vi "XYZ-BC.vi"(5 "加速度":dbl=600.0, 7 "最高速":dbl=1250.0, 8 "Error In":errorcluster, 9 "校正微動位置":enum16{"雙邊", "オ", "右", "相反"}(ring), 11 "X-Y-Z移動":dbl[](array[numeric])=[0.0, 0.0, 0.0]) -> (0 "Error Out":errorcluster)   [LabVIEW 2019]
uses:
  <vilib>/Platform/TimedLoop/XDataNode/timing_clust.ctl
  <vilib>/Platform/TimedLoop/XDataNode/nitl_modes.ctl
  <vilib>/Platform/TimedLoop/XDataNode/wakeup.ctl
  <vilib>/platform/TimedLoop/XDataNode/XDataNode.xnode
  <vilib>/Platform/TimedLoop/XDataNode/XDNodeRunTimeDep.lvlib
panel:
  in  "Stop":bool
  out "三角形?":bool
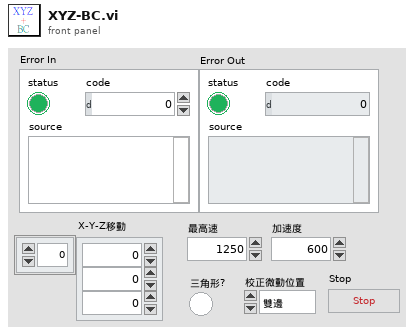
[diagram p1: front panel]
types:
  T1 = typedef "XDNodeRunTimeDep.lvlib/timing_clust.ctl" = cluster{"Expected End [f-1]":u64, "Actual End [f-1]":u64, "Finished Late? [f-1]":bool, "Expected End [i-1]":u64, "Actual End [i-1]":u64, "Finished Late? [i-1]":bool, "Expected Start [i]":u64, "Actual Start [i]":u64, "Expected Start [f]":u64, "Actual Start [f]":u64, "Source Name":string, "Structure Name":string, "Period":i64, "Deadline":i64, "Offset":i64, "Start":i64, "Priority":i32, "Timeout":i32, "Mode":T2, "Wakeup Reason":T3, "Error":errorcluster, "Source Type":string, "Secondary Source Type":string, "Global End Time":u64, "Global Start Time":u64, "Frame Duration":u64, "Iteration Duration":u64, "Assigned CPU":i32, "I/O Scan Engine Mode":u32}
  T2 = typedef "XDNodeRunTimeDep.lvlib/nitl_modes.ctl" = enum32{"No Change", "Process missed periods, maintain original phase", "Discard missed periods, maintain original phase", "Process missed periods, ignore original phase", "Discard missed periods, ignore original phase"}
  T3 = typedef "XDNodeRunTimeDep.lvlib/wakeup.ctl" = enum32{"Normal", "Aborted", "Asynchronous wakeup", "Timing source error", "Timed loop error", "Timeout"}
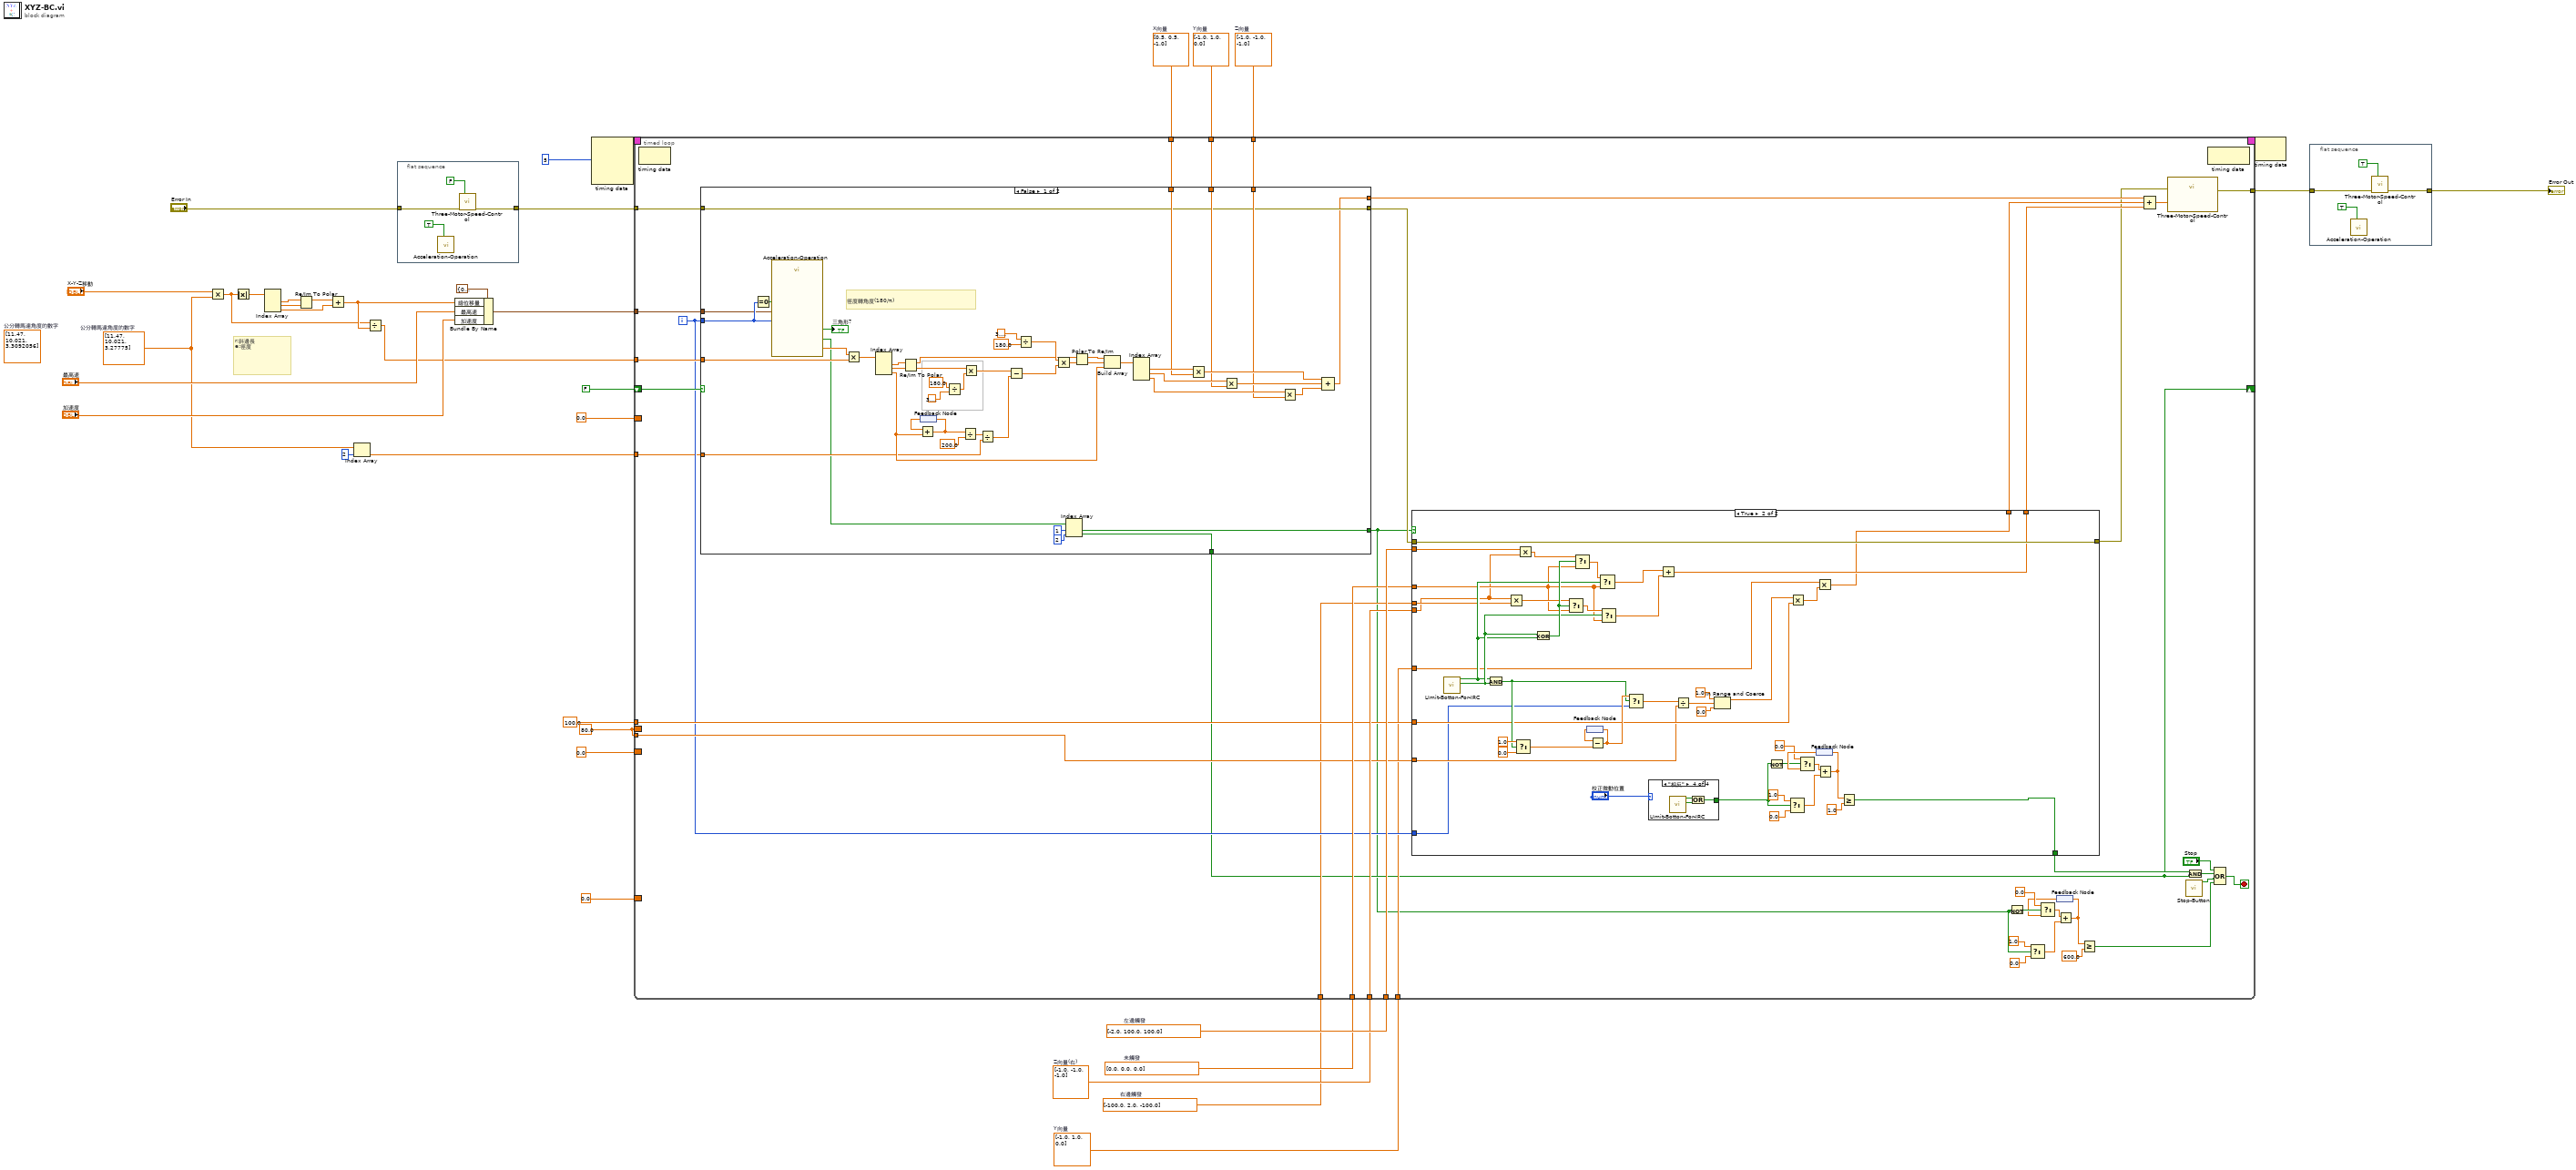
[diagram p0: block diagram]
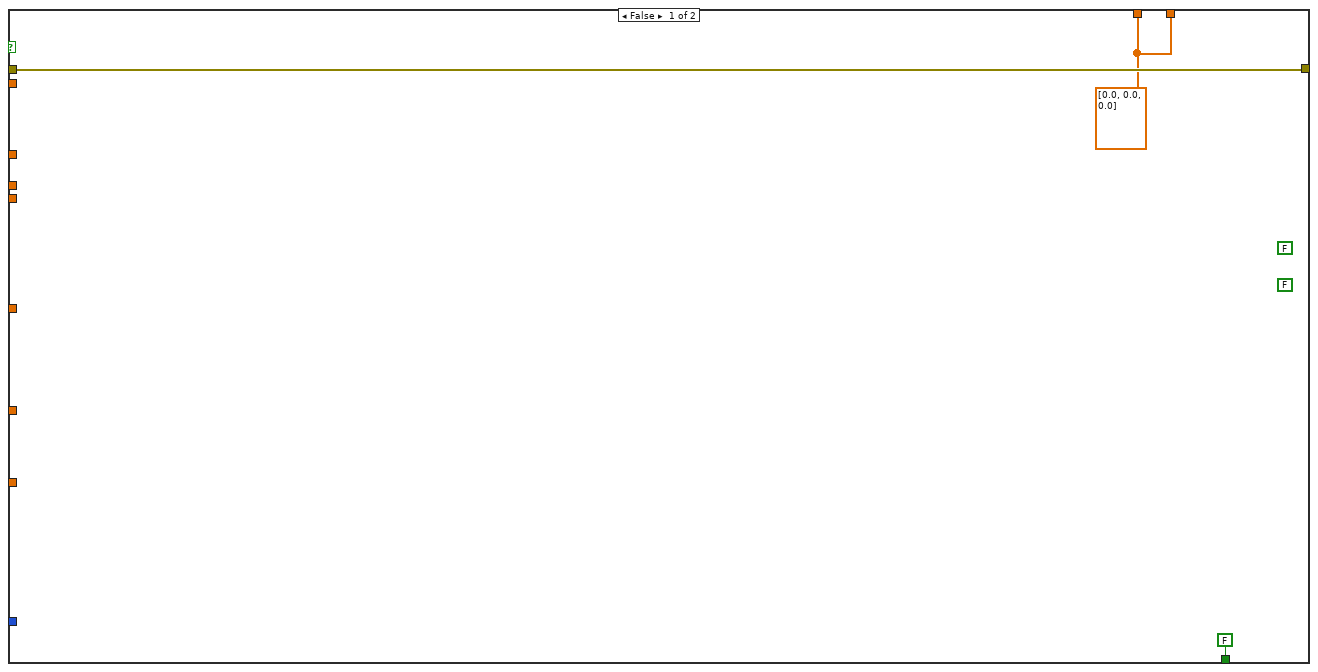
[diagram p2: hidden frame]
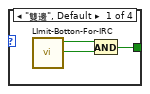
[diagram p3: hidden frame]
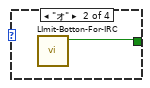
[diagram p4: hidden frame]
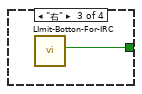
[diagram p5: hidden frame]
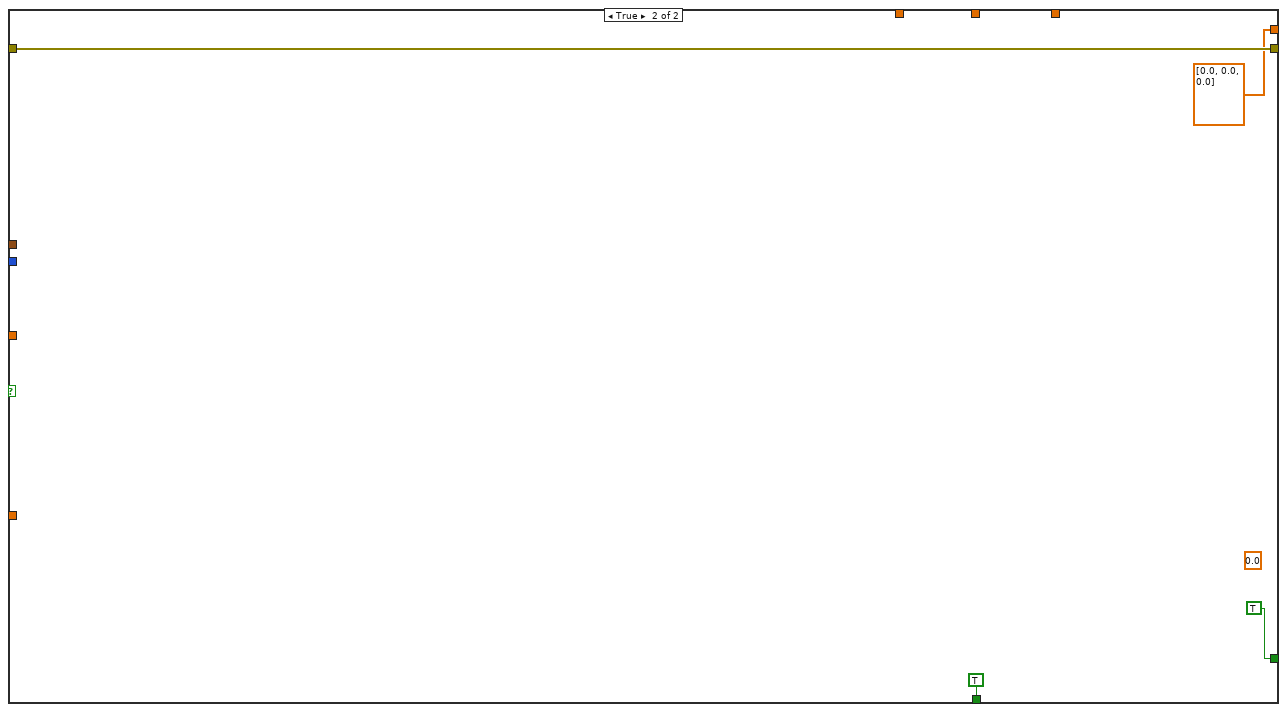
[diagram p6: hidden frame]
diagram:
  w11 = 80.0
  w14 = dbl[] [0.0, 0.0, 0.0]  # 未觸發
  w10 = dbl[] [-100.0, 2.0, -100.0]  # 右邊觸發
  w15 = dbl[] [-2.0, 100.0, 100.0]  # 左邊觸發
  w13 = dbl[] [-1.0, -1.0, -1.0]  # Z向量(右)
  w9 = dbl[] [-1.0, 1.0, 0.0]  # Y向量
  w18 = dbl[] [-1.0, -1.0, -1.0]  # Z向量
  w19 = dbl[] [-1.0, 1.0, 0.0]  # Y向量
  w20 = dbl[] [0.5, 0.5, -1.0]  # X向量
  (unwired) dbl[] [11.47, 10.021, 3.3092056]  # 公分轉馬達角度的數字
  w27 = dbl[] [11.47, 10.021, 3.27775]  # 公分轉馬達角度的數字
  # "r:斜邊長\ne:徑度"
  n1 = Multiply(x="X-Y-Z移動", y=w27) -> (x*y=w28:dbl[])
  n2 = Absolute Value(x=w28) -> (abs(x)=w36:dbl[])
  n3 = Index Array(array=w36) -> (element #1=w32:dbl, element #2=w37:dbl, element #3=w33:dbl)  [unwired: 3 in]
  n4 = Re/Im To Polar(2:w37, 3:w32) -> (1:w34:dbl)  [unwired: 1 out]
  n5 = Add(x=w34, y=w33) -> (x+y=w29:dbl)
  n6 = Index Array(array=w27, index=2) -> (element=w25:dbl)
  n7 = Divide(x=w28, y=w29) -> (x/y=w22:dbl[])
  n8 = flat-sequence {
    tunnel: "Error In" -> [w40]
    tunnel: [w39] -> w21
    frame #0 {
      n9 = call "Acceleration-Operation.vi"("Reset"=TRUE) -> ()  [unwired: 8 in, 3 out]
      n10 = call "Three-Motor-Speed-Control.vi"("Reset"=FALSE, "Error In"=w40) -> ("Error Out"=w39:errorcluster)  [unwired: 9 in]
    }
  }
  n11 = Bundle By Name(cluster=cluster{"總位移量":dbl, "最高速":dbl, "加速度":dbl} {"總位移量"=0.0, "最高速"=0.0, "加速度"=0.0} ("計算設置"), "總位移量"=w29, "最高速"="最高速", "加速度"="加速度") -> (w24:cluster{"總位移量":dbl, "最高速":dbl, "加速度":dbl})
  n12 = node-c288(i64 5 ("Period")) -> (w7:T1)  [unwired: 3 in]
  n13 = timed-loop {
    border: 0.0 -> [_]
    tunnel: w25 -> [w53]
    tunnel: w24 -> [w81]
    tunnel: w22 -> [w80]
    tunnel: w21 -> [w79]
    tunnel: w20 -> [w78]
    tunnel: w19 -> [w77]
    tunnel: w18 -> [w76]
    shift-right: [w54] -> _
    shift-left: FALSE -> [w75]
    border: 0.0 -> [_]
    border: w11 -> [_]
    tunnel: w15 -> [w70]
    tunnel: w14 -> [w69]
    tunnel: w13 -> [w68]
    tunnel: 100.0 -> [w67]
    tunnel: w11 -> [w66]
    tunnel: w10 -> [w64]
    tunnel: w9 -> [w63]
    tunnel: [w57] -> w8
    timing: w7 -> [_]
    timing-out: [_] -> w6
    border: 0.0 -> [_]
    i -> [w65]
    stop <- w74 stop-if-true
    n14 = node-c288() -> ()  [unwired: 1 in, 1 out]
    n15 = case shown="False" w75 {
      tunnel: w65 -> [w152 _]
      tunnel: w53 -> [w151 _]
      tunnel: w81 -> [w150 _]
      tunnel: w80 -> [w149 _]
      tunnel: w79 -> [w142 w186]
      tunnel: w78 -> [w148 _]
      tunnel: w77 -> [w147 _]
      tunnel: w76 -> [w146 _]
      tunnel: [w139 TRUE] -> w43
      tunnel: [w140 TRUE] -> w54
      tunnel: [w142 w186] -> w62
      tunnel: [w141 dbl[] [0.0, 0.0, 0.0]] -> w58
      frame False {
        # "徑度轉角度(180/π)"
        n16 = Equal To 0?(x=w152) -> (x = 0?=w183:bool)
        n17 = call "Acceleration-Operation.vi"("Reset"=w183, "迴圈( I )"=w152, "計算設置"=w150) -> ("完成?"=w145:bool[], "速度"=w184:dbl, "三角形?"=→"三角形?":bool)  [unwired: 6 in]
        n18 = Multiply(x=w184, y=w149) -> (x*y=w181:dbl[])
        n19 = Index Array(array=w181) -> (element #1=w180:dbl, element #2=w179:dbl, element #3=w162:dbl)  [unwired: 3 in]
        n20 = Re/Im To Polar(2:w179, 3:w180) -> (0:w178:dbl, 1:w165:dbl)
        n21 = feedback #1() -> (w174:dbl)
        n22 = Add(x=w174, y=w162) -> (x+y=w173:dbl)
        n23 = feedback-in #1(w173) -> ()
        n24 = Divide(x=180.0, y=3.141592653589793) -> (x/y=w175:dbl)
        n25 = Divide(x=w173, y=200.0) -> (x/y=w154:dbl)
        n26 = Multiply(x=w178, y=w175) -> (x*y=w171:dbl)
        n27 = Divide(x=w154, y=w151) -> (x/y=w153:dbl)
        n28 = Subtract(x=w171, y=w153) -> (x-y=w167:dbl)
        n29 = Divide(x=3.141592653589793, y=180.0 ("x")) -> (x/y=w168:dbl)
        n30 = Multiply(x=w168, y=w167) -> (x*y=w166:dbl)
        n31 = Index Array(array=w145, index #1=1 ("index"), index #2=2 ("index")) -> (element #1=w139:bool, element #2=w140:bool)
        n32 = Polar To Re/Im(2:w166, 3:w165) -> (0:w163:dbl, 1:w164:dbl)
        n33 = Build Array(w164, w163, w162) -> (w161:dbl[])
        n34 = Index Array(array=w161) -> (element #1=w160:dbl, element #2=w159:dbl, element #3=w158:dbl)  [unwired: 3 in]
        n35 = Multiply(x=w160, y=w148) -> (x*y=w157:dbl[])
        n36 = Multiply(x=w159, y=w147) -> (x*y=w156:dbl[])
        n37 = Multiply(x=w158, y=w146) -> (x*y=w155:dbl[])
        n38 = Compound Arithmetic op=ADD(w157, w156, w155) -> (w141:dbl[])
      }
      frame True {
        (unwired) 0.0
      }
    }
    n39 = case shown="True" w43 {
      tunnel: [FALSE w87] -> w71
      tunnel: w70 -> [_ w98]
      tunnel: w69 -> [_ w97]
      tunnel: w68 -> [_ w92]
      tunnel: w67 -> [_ w96]
      tunnel: w66 -> [_ w95]
      tunnel: w65 -> [_ w94]
      tunnel: w64 -> [_ w93]
      tunnel: w63 -> [_ w91]
      tunnel: w62 -> [w86 w90]
      tunnel: [w86 w90] -> w55
      tunnel: [w84 w89] -> w60
      tunnel: [w84 w88] -> w59
      frame False {
        (unwired) FALSE
        (unwired) FALSE
        w84 = dbl[] [0.0, 0.0, 0.0]
      }
      frame True {
        n40 = call "LImit-Botton-For-IRC.vi"() -> ("微動觸發(右)?"=w111:bool, "微動觸發(左)?"=w110:bool)  [unwired: 9 in, 1 out]
        n41 = And(x=w110, y=w111) -> (x .and. y?=w116:bool)
        n42 = Multiply(x=w92, y=w93) -> (x*y=w112:dbl[])
        n43 = Select(t=1.0, s=w116, f=0.0) -> (s? t:f=w129:dbl)
        n44 = Multiply(x=w98, y=w92) -> (x*y=w113:dbl[])
        n45 = Exclusive Or(1:w110, 2:w111) -> (0:w114:bool)
        n46 = Select(t=w112, s=w114, f=w97) -> (s? t:f=w115:dbl[])
        n47 = Select(t=w113, s=w114, f=w97) -> (s? t:f=w117:dbl[])
        n48 = feedback #2() -> (w128:dbl)
        n49 = Subtract(x=w128, y=w129) -> (x-y=w127:dbl)
        n50 = feedback-in #2(w127) -> ()
        n51 = Select(t=w117, s=w110, f=w97) -> (s? t:f=w119:dbl[])
        n52 = Select(t=w115, s=w111, f=w97) -> (s? t:f=w118:dbl[])
        n53 = Select(t=w127, s=w116, f=w94) -> (s? t:f=w126:dbl)
        n54 = case shown="\"相反\"" "校正微動位置" {
          tunnel: [w131 w134 w135 w136] -> w99
          frame "雙邊", Default {
            n55 = call "LImit-Botton-For-IRC.vi"() -> ("微動觸發(右)?"=w132:bool, "微動觸發(左)?"=w133:bool)  [unwired: 9 in, 1 out]
            n56 = And(x=w133, y=w132) -> (x .and. y?=w131:bool)
          }
          frame "オ" {
            n57 = call "LImit-Botton-For-IRC.vi"() -> ("微動觸發(左)?"=w134:bool)  [unwired: 9 in, 2 out]
          }
          frame "右" {
            n58 = call "LImit-Botton-For-IRC.vi"() -> ("微動觸發(右)?"=w135:bool)  [unwired: 9 in, 2 out]
          }
          frame "相反" {
            n59 = call "LImit-Botton-For-IRC.vi"() -> ("微動觸發(右)?"=w137:bool, "微動觸發(左)?"=w138:bool)  [unwired: 9 in, 1 out]
            n60 = Or(x=w138, y=w137) -> (x .or. y?=w136:bool)
          }
        }
        n61 = Add(x=w119, y=w118) -> (x+y=w89:dbl[])
        n62 = Divide(x=w126, y=w95) -> (x/y=w124:dbl)
        n63 = In Range and Coerce(upper limit=1.0, x=w124, lower limit=0.0) -> (coerced(x)=w121:dbl)  [unwired: 1 out]
        n64 = Not(x=w99) -> (.not. x?=w104:bool)
        n65 = Select(t=1.0, s=w99, f=0.0) -> (s? t:f=w106:dbl)
        n66 = Multiply(x=w121, y=w96) -> (x*y=w120:dbl)
        n67 = feedback #3() -> (w105:dbl)
        n68 = Select(t=0.0, s=w104, f=w105) -> (s? t:f=w102:dbl)
        n69 = Multiply(x=w91, y=w120) -> (x*y=w88:dbl[])
        n70 = Add(x=w102, y=w106) -> (x+y=w101:dbl)
        n71 = feedback-in #3(w101) -> ()
        n72 = Greater Or Equal?(x=w101, y=1.0) -> (x >= y?=w87:bool)
      }
    }
    n73 = Not(x=w43) -> (.not. x?=w48:bool)
    n74 = Select(t=1.0, s=w43, f=0.0) -> (s? t:f=w46:dbl)
    n75 = feedback #4() -> (w47:dbl)
    n76 = Select(t=0.0, s=w48, f=w47) -> (s? t:f=w50:dbl)
    n77 = Add(x=w50, y=w46) -> (x+y=w51:dbl)
    n78 = feedback-in #4(w51) -> ()
    n79 = Greater Or Equal?(x=w51, y=600.0) -> (x >= y?=w42:bool)
    n80 = Compound Arithmetic op=ADD(w58, w59, w60) -> (w61:dbl[])
    n81 = call "Three-Motor-Speed-Control.vi"("Error In"=w55, "速度(秒/度)"=w61) -> ("Error Out"=w57:errorcluster)  [unwired: 9 in]
    n82 = call "Stop-Button.vi"() -> ("顯示按下?"=w73:bool)  [unwired: 10 in, 1 out]
    n83 = And(x=w71, y=w54) -> (x .and. y?=w72:bool)
    n84 = node-c288() -> ()  [unwired: 1 in, 1 out]
    n85 = Compound Arithmetic op=OR("Stop", w72, w73, w42) -> (w74:bool)
  }
  n86 = node-c288(w6) -> ()  [unwired: 1 out]
  n87 = flat-sequence {
    tunnel: w8 -> [w191]
    tunnel: [w190] -> w3
    frame #0 {
      n88 = call "Acceleration-Operation.vi"("Reset"=TRUE) -> ()  [unwired: 8 in, 3 out]
      n89 = call "Three-Motor-Speed-Control.vi"("Reset"=TRUE, "Error In"=w191) -> ("Error Out"=w190:errorcluster)  [unwired: 9 in]
    }
  }
  "Error Out" <- w3
